vi "Write_spectra_to_FLASH.vi"() -> ()   [LabVIEW 2022 SP3]
uses:
  <vilib>/Utility/file.llb/Read From Spreadsheet File (DBL).vi
  adcDLL_0001.dll
panel:
  out "cycle":i32
  out "Waveform Graph 2":u8[](graph)
  out "first row":dbl[](array[numeric]) format="%0.3f"
  out "Array":u8[](array[numeric])
  out "output array":u8[](array[numeric]) format="%x"
  in  "DevDet":i32=1
  in  "address_flash":u16=1
  in  "address_buffer":u16=4
  out "size(s)":i32
  out "Waveform Graph":u16[](graph)
  out "initialized array":u8[](array[numeric])
  out "Spectra":u16[](array[numeric])
  out "Input Report":u8[](array[numeric])
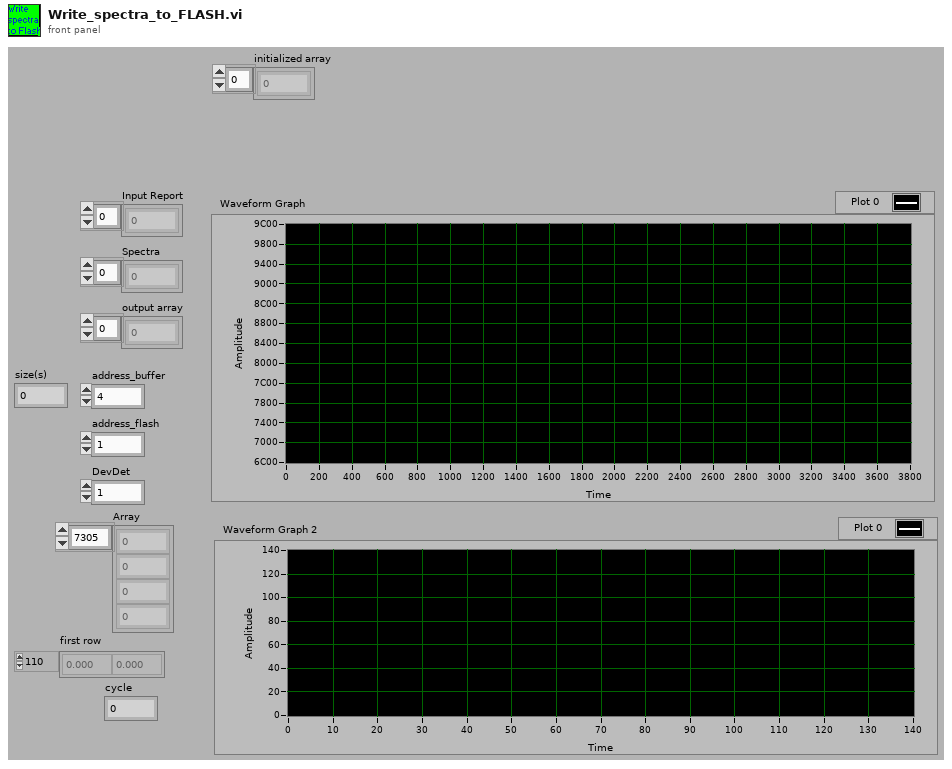
[diagram p1: front panel]
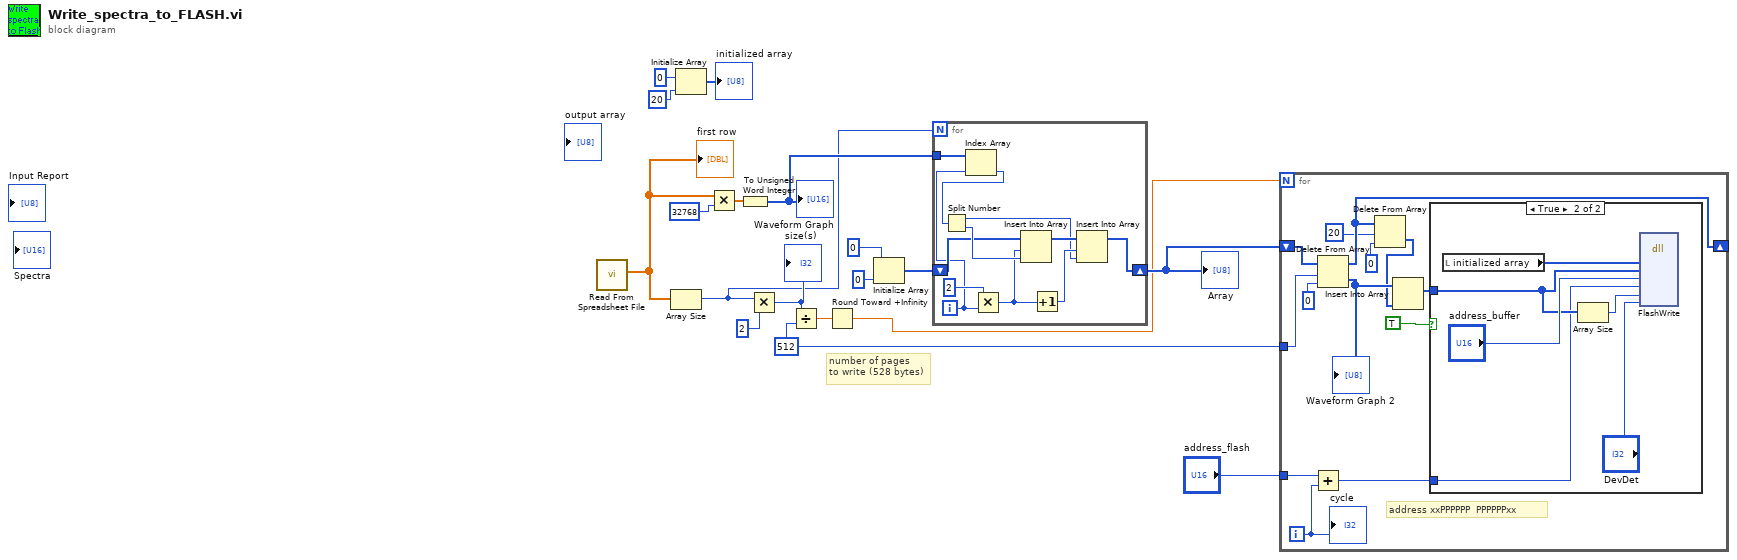
[diagram p0: block diagram]
diagram:
  w1 = 512
  # "number of pages\nto write (528 bytes)"
  n1 = call-poly <vilib>:"Read From Spreadsheet File.vi"() -> ("first row"=w10:dbl[])  [unwired: 7 in, 4 out]
  "first row" <- w10
  n2 = Array Size(array=w10) -> (size(s)=w5:i32)
  n3 = Initialize Array(u8 0 ("element"), 20 ("dimension size")) -> (→"initialized array":u8[])
  n4 = Multiply(x=w10, y=u16 32768) -> (x*y=w11:dbl[])
  n5 = To Unsigned Word Integer(number=w11) -> (unsigned 16bit integer=w9:u16[])
  "Waveform Graph" <- w9
  n6 = Multiply(x=w5, y=2) -> (x*y=w14:i32)
  "size(s)" <- w14
  n7 = Divide(x=w14, y=w1) -> (x/y=w15:dbl)
  n8 = Round Toward +Infinity(x=w15) -> (ceil(x): smallest int >= x=w2:dbl)
  n9 = Initialize Array(u8 0 ("element"), 0 ("dimension size")) -> (w6:u8[])
  n10 = for {
    N: w5 -> [_]
    tunnel: w9 -> [w21]
    shift-right: [w22] -> w3
    shift-left: w6 -> [w27]
    i -> [w20]
    n11 = Index Array(array=w21, index=w20) -> (element=w19:u16)
    n12 = Split Number(x=w19) -> (hi(x)=w23:u8, lo(x)=w28:u8)
    n13 = Multiply(x=2, y=w20) -> (x*y=w25:i32)
    n14 = Insert Into Array(array=w27, index=w25, new element=w28) -> (w26:u8[])
    n15 = Increment(x=w25) -> (x+1=w24:i32)
    n16 = Insert Into Array(array=w26, index=w24, new element=w23) -> (w22:u8[])
  }
  "Array" <- w3
  n17 = for {
    N: w2 -> [_]
    shift-right: [w33] -> _
    shift-left: w3 -> [w41]
    tunnel: w1 -> [w40]
    tunnel: "address_flash" -> [w38]
    i -> [w37]
    # "address xxPPPPPP  PPPPPPxx"
    n18 = Add(x=w38, y=w37) -> (x+y=w36:i32)
    n19 = Delete From Array(array=w41, length=w40, index=0) -> (deleted portion=w34:u8[], array with subset deleted=w33:u8[])
    "Waveform Graph 2" <- w34
    n20 = Delete From Array(array=w33, length=20, index=0) -> (deleted portion=w32:u8[])  [unwired: 1 out]
    n21 = Insert Into Array(array=w34, new element=w32) -> (w35:u8[])  [unwired: 1 in]
    n22 = case shown="True" TRUE {
      tunnel: w35 -> [_ w44]
      tunnel: w36 -> [_ w43]
      frame False {
      }
      frame True {
        n23 = local read "initialized array"() -> (w45:u8[])
        n24 = Array Size(array=w44) -> (size(s)=w46:i32)
        n25 = dll-call lib="D:/LabVIEWSuite_64_OS/Spectrometers/ASEQ LR1/adcDLL_0001.dll" fn="FlashWrite"("OutputReport1"=w45, "OutputData1"=w44, "address_buffer"="address_buffer", "address_flash"=w43, "length"=w46, "DevDet"="DevDet") -> ()  [unwired: 10 in, 2 out]
      }
    }
    "cycle" <- w37
  }
